vi "Build Graph Buffer.vi"(10 "Graph Buffer Size":i32, 11 "Channel Count":i32) -> (3 "Graph Buffer out":cluster{dbl[], dbl[]}[](array[cluster]))   [LabVIEW 2012, in "Workspace MultiY Graph.lvlib"]
doc: "Build the graph buffer based on the graph buffer size and channel count."
uses:
  Workspace MultiY Graph.lvlib
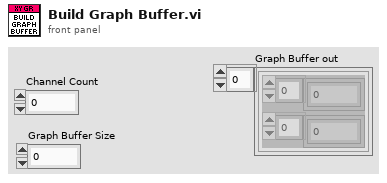
[diagram p1: front panel]
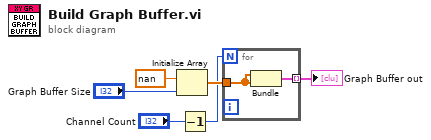
[diagram p0: block diagram]
diagram:
  n1 = Initialize Array(nan ("element"), "Graph Buffer Size") -> (w4:dbl[])
  n2 = Decrement(x="Channel Count") -> (x-1=w2:i32)
  n3 = for {
    N: w2 -> [_]
    tunnel: w4 -> [w8]
    tunnel: [w7] -> w6 mode=indexing
    n4 = Bundle(w8, w8) -> (w7:cluster{dbl[], dbl[]})  [unwired: 1 in]
  }
  "Graph Buffer out" <- w6
